vi "bon format de produit.vi"(1 "Chaîne":string="12-216C-04521_EQIFIL_417mA_14-4Ohm") -> (0 "Chaîne 2":string="12-216C-04521 EQIFIL 417mA 14.4ohm")   [LabVIEW 2020]
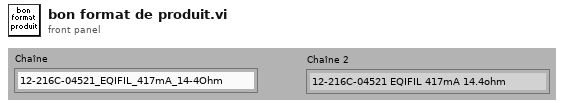
[diagram p1: front panel]
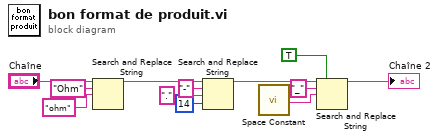
[diagram p0: block diagram]
diagram:
  n1 = Search and Replace String(input string="Chaîne", search string="Ohm" ("chaîne recherchée"), replace string="ohm" ("chaîne recherchée")) -> (result string=w11:string)  [unwired: 5 in, 3 out]
  n2 = Search and Replace String(input string=w11, search string="-" ("chaîne recherchée"), replace string="." ("chaîne de remplacement (\"\")"), offset=14 ("offset (0)")) -> (result string=w10:string)  [unwired: 4 in, 3 out]
  n3 = call <vilib>:"Space Constant.vi"() -> ("String"=w4:string)
  n4 = Search and Replace String(replace all?=TRUE ("tout remplacer ? (F)"), input string=w10, search string="_" ("chaîne recherchée"), replace string=w4) -> (result string=→"Chaîne 2":string)  [unwired: 4 in, 3 out]
